vi "Position Terminals.vi"(6 "Terminal Configs":T4[](array[typedef]), 8 "error in (no error)":errorcluster, 11 "Refs in":T1) -> (0 "error out":errorcluster, 2 "Grouped Terminals":T2, 3 "Refs":T1)   [LabVIEW 2020, in "FlexBlocks.lvlib"]
uses:
  FlexBlocks.lvlib
  Terminal Direction.ctl
  Value Mode.ctl
  Special Terminal.ctl
  Type Descriptor.ctl
  Terminal Mode.ctl
  Terminal Config.ctl
  Terminal Group.ctl
  Grouped Terminals.ctl
  Scripting Refs.ctl
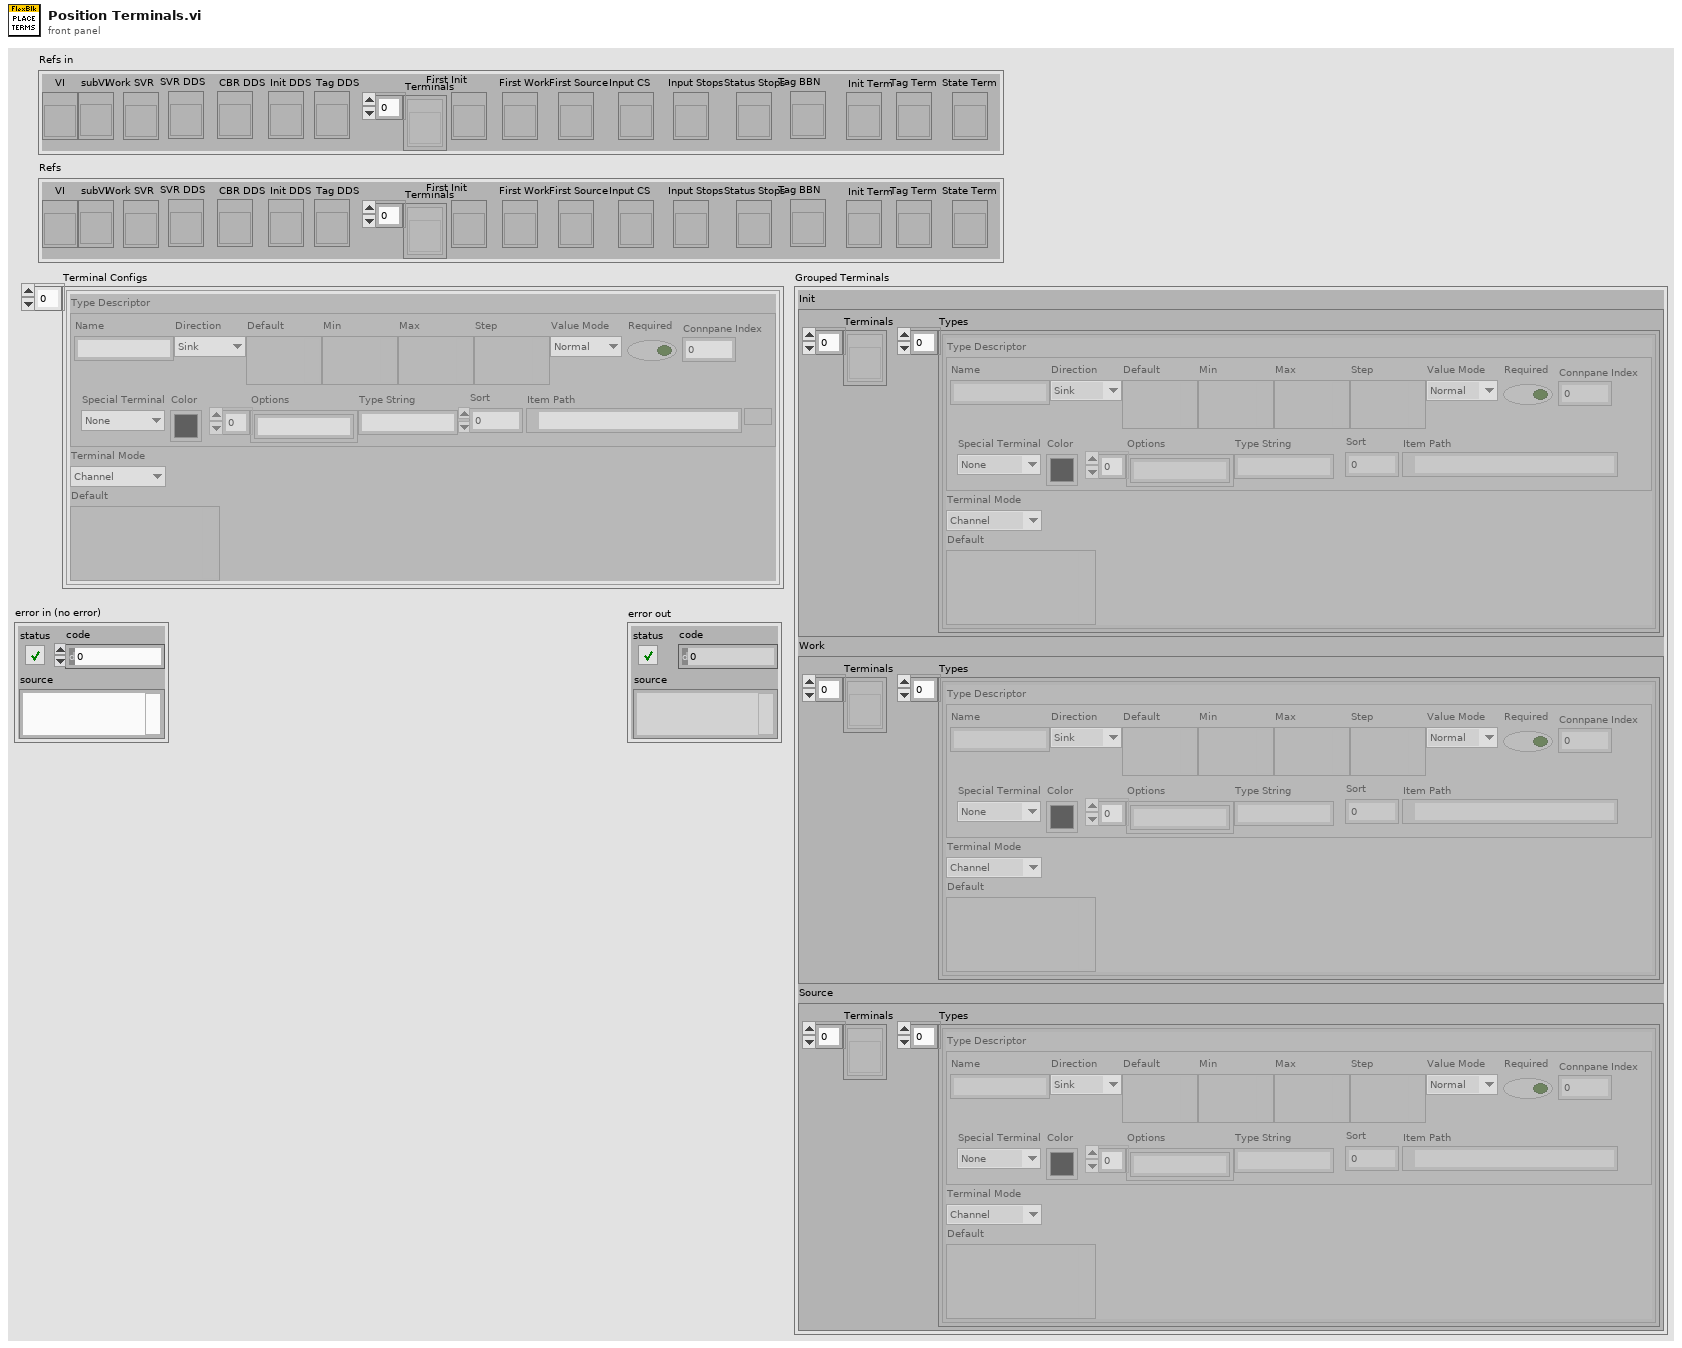
[diagram p1: front panel]
types:
  T1 = typedef "FlexBlocks.lvlib/Scripting Refs.ctl" = cluster{"VI":refnum<vi>, "subVI":refnum<vi>, "Work SVR":refnum<vi>, "SVR DDS":refnum<vi>, "CBR DDS":refnum<vi>, "Init DDS":refnum<vi>, "Tag DDS":refnum<vi>, "Terminals":refnum<vi>[], "First Init":refnum<vi>, "First Work":refnum<vi>, "First Source":refnum<vi>, "Input CS":refnum<vi>, "Input Stops":refnum<vi>, "Status Stops":refnum<vi>, "Tag BBN":refnum<vi>, "Init Term":refnum<vi>, "Tag Term":refnum<vi>, "State Term":refnum<vi>}
  T2 = typedef "FlexBlocks.lvlib/Grouped Terminals.ctl" = cluster{"Init":T3, "Work":T3, "Source":T3}
  T3 = typedef "FlexBlocks.lvlib/Terminal Group.ctl" = cluster{"Terminals":refnum<vi>[], "Types":T4[]}
  T4 = typedef "FlexBlocks.lvlib/Terminal Config.ctl" = cluster{"Type Descriptor":T5, "Terminal Mode":T9, "Default":variant}
  T5 = typedef "FlexBlocks.lvlib/Type Descriptor.ctl" = cluster{"Name":string, "Direction":T6, "Default":variant, "Min":variant, "Max":variant, "Step":variant, "Value Mode":T7, "Required":bool, "Connpane Index":i32, "Special Terminal":T8, "Color":u32, "Options":string[], "Type String":string, "Sort":i32, "Item Path":path}
  T6 = typedef "FlexBlocks.lvlib/Terminal Direction.ctl" = enum16{"Sink", "Source"}
  T7 = typedef "FlexBlocks.lvlib/Value Mode.ctl" = enum16{"Normal", "Range", "Select"}
  T8 = typedef "FlexBlocks.lvlib/Special Terminal.ctl" = enum16{"None", "Action", "Init", "Tag", "State in", "State out", "Error"}
  T9 = typedef "FlexBlocks.lvlib/Terminal Mode.ctl" = enum16{"Channel", "Config", "Value", "Control Ref"}
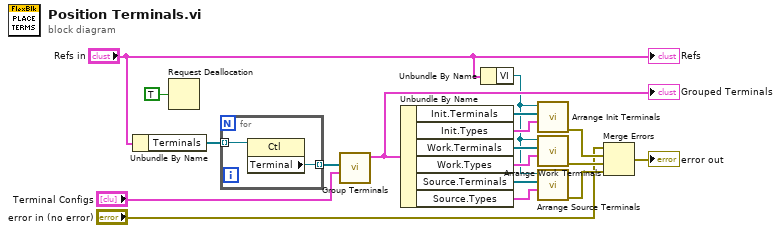
[diagram p0: block diagram]
diagram:
  n1 = Unbundle By Name("Refs in") -> ("Terminals"=w3:refnum<vi>[])
  n2 = Request Deallocation(TRUE ("flag")) -> ()
  n3 = for {
    tunnel: w3 -> [w20] mode=indexing
    tunnel: [w19] -> w17 mode=indexing
    n4 = property class="Ctl"(reference=w20) -> ("Terminal"=w19:refnum<vi>)  [unwired: 1 in, 2 out]
  }
  n5 = call "Group Terminals.vi"("Terminal Configs"="Terminal Configs", "Terminals"=w17) -> ("Grouped Terminals"=w10:T2)  [unwired: 9 in]
  "Grouped Terminals" <- w10
  n6 = Unbundle By Name(w10) -> ("Init.Terminals"=w9:refnum<vi>[], "Init.Types"=w6:T4[], "Work.Terminals"=w7:refnum<vi>[], "Work.Types"=w5:T4[], "Source.Terminals"=w8:refnum<vi>[], "Source.Types"=w4:T4[])
  n7 = Unbundle By Name("Refs in") -> ("VI"=w1:refnum<vi>)
  n8 = call "Arrange Init Terminals.vi"("Init Types"=w6, "Init Terminals"=w9, "VI"=w1) -> ("error out"=w15:errorcluster)  [unwired: 8 in]
  n9 = call "Arrange Work Terminals.vi"("Work Types"=w5, "Work Terminals"=w7, "VI"=w1) -> ("error out"=w14:errorcluster)  [unwired: 8 in]
  n10 = call "Arrange Source Terminals.vi"("Source Types"=w4, "Source Terminals"=w8, "VI"=w1) -> ("error out"=w13:errorcluster)  [unwired: 8 in]
  n11 = Merge Errors("error in (no error)", w15, w14, w13) -> (→"error out":errorcluster)
  "Refs" <- "Refs in"
